vi "Close.vi"(8 "error in (no error)":errorcluster, 11 "Normal Log in":refnum<class "Normal Log.lvclass">) -> (0 "error out":errorcluster)   [LabVIEW 2020, in "Normal Log.lvlib" / "Normal Log.lvclass"]
uses:
  Normal Log.lvclass
  <vilib>/ActorFramework/Stop Msg/Stop Msg.lvclass
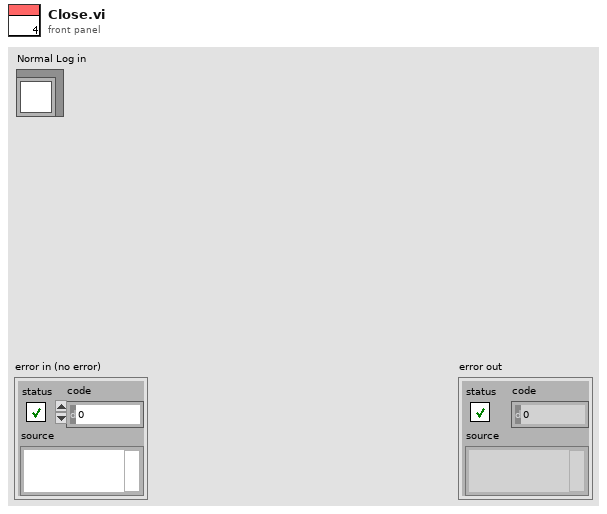
[diagram p1: front panel]
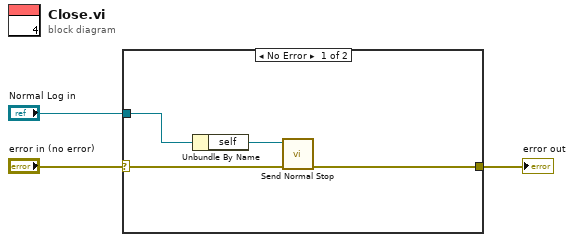
[diagram p0: block diagram]
diagram:
  n1 = case shown="No Error" "error in (no error)" {
    selector: "error in (no error)" -> [w6 w8]
    tunnel: "Normal Log in" -> [w7 _]
    tunnel: [w4 w8] -> w1
    frame No Error {
      n2 = Unbundle By Name(w7) -> ("self"=w5:refnum<class "Message Enqueuer.lvclass">)
      n3 = call <vilib>:"Send Normal Stop.vi"("error in (no error)"=w6, "Message Enqueuer"=w5) -> ("error out"=w4:errorcluster)  [unwired: 9 in]
    }
    frame Error {
    }
  }
  "error out" <- w1
